vi "Decimator Function.vi"(6 "Max Size (10K)":i32=10000, 9 "Decimation #":i32, 10 "Input Y values New":dbl[](array[numeric]), 11 "Input Y values Old":dbl[](array[numeric])) -> (3 "Output Y Values":dbl[](array[numeric]))   [LabVIEW 2014]
panel:
  # "Decimator Function"
  # "Inputs"
  # "Outputs"
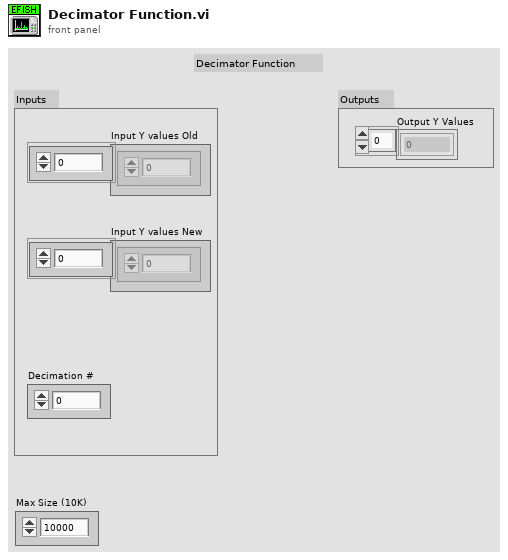
[diagram p1: front panel]
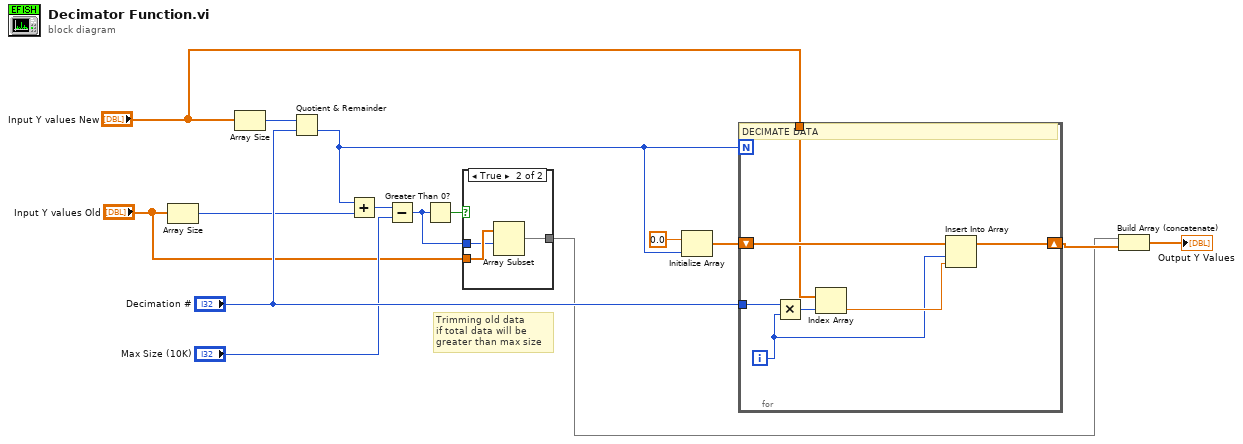
[diagram p0: block diagram]
diagram:
  # "Trimming old data\nif total data will be \ngreater than max size"
  n1 = Array Size(array="Input Y values Old") -> (size(s)=w12:i32)
  n2 = Array Size(array="Input Y values New") -> (size(s)=w14:i32)
  n3 = Quotient & Remainder(x=w14, y="Decimation #") -> (floor(x/y)=w11:i32)  [unwired: 1 out]
  n4 = Add(x=w11, y=w12) -> (x+y=w10:i32)
  n5 = Subtract(x=w10, y="Max Size (10K)") -> (x-y=w7:i32)
  n6 = Greater Than 0?(x=w7) -> (x > 0?=w8:bool)
  n7 = case shown="True" w8 {
    tunnel: "Input Y values Old" -> [w16 w19]
    tunnel: w7 -> [_ w18]
    tunnel: [w16 w17] -> w1
    frame False {
    }
    frame True {
      n8 = Array Subset(array=w19, index=w18) -> (w17:dbl[])  [unwired: 1 in]
    }
  }
  n9 = Initialize Array(0.0 ("Numeric Control"), w11) -> (w4:dbl[])
  n10 = for {
    N: w11 -> [_]
    shift-right: [w23] -> w3
    shift-left: w4 -> [w24]
    tunnel: "Decimation #" -> [w26]
    tunnel: "Input Y values New" -> [w22]
    i -> [w20]
    # "DECIMATE DATA"
    n11 = Multiply(x=w26, y=w20) -> (x*y=w25:i32)
    n12 = Index Array(array=w22, index=w25) -> (element=w21:dbl)
    n13 = Insert Into Array(array=w24, index=w20, new element=w21) -> (w23:dbl[])
  }
  n14 = Build Array (concatenate)(w1, w3) -> (→"Output Y Values":dbl[])
